vi "GUI Write Sequence Item Status.vi"(7 "status label":string="stat2", 8 "error in":errorcluster, 11 "sequence item":T1) -> (0 "error out":errorcluster, 3 "sequence item (copy)":T1)   [LabVIEW 2018]
doc: "Updates measurement status for each sequence item. Can generate error, but will exdcute even with input error."
uses:
  Meas Sequence Item.ctl
  Meas Sampling Configuration.ctl
  adc/ADC Trig Config.ctl
  adc/ADC Trig Mode Source.ctl
  adc/ADC Trig Coupling.ctl
  adc/ADC Trig Slope.ctl
  processing/QWTB/Meas Proc QWTB Algorithm Parameter Data.ctl
  varilib/SGUI Assign Multiple Strings With Tags By Label.vi
  varilib/varilib.lvlib
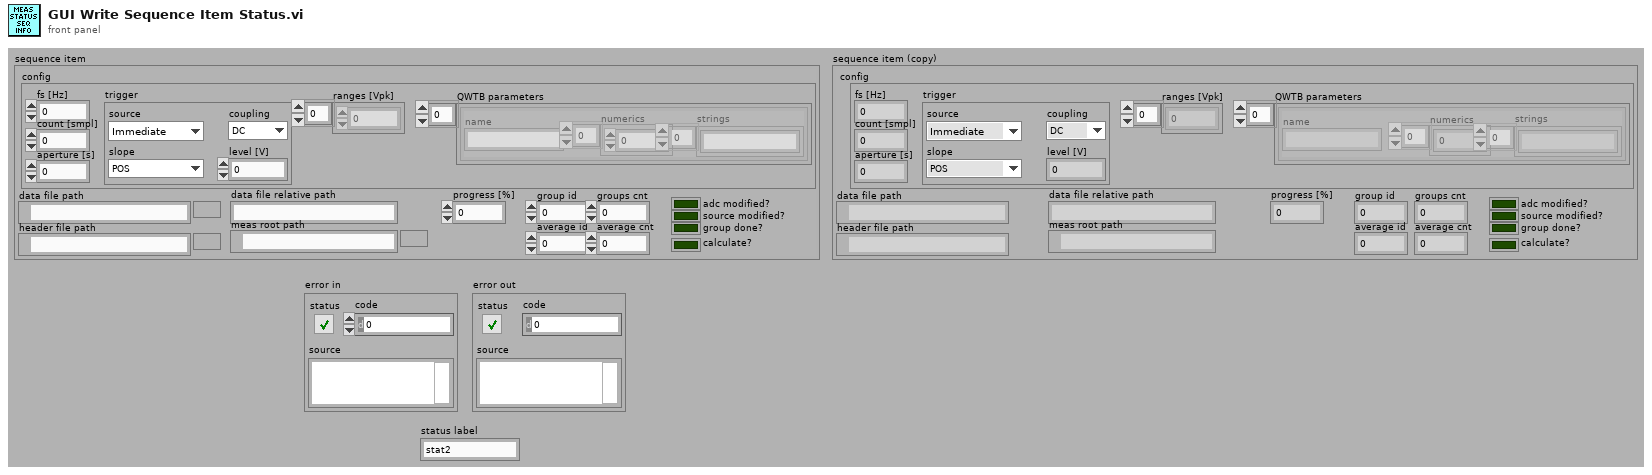
[diagram p1: front panel]
types:
  T1 = typedef "Meas Sequence Item.ctl" = cluster{"config":T2, "data file path":path, "header file path":path, "group id":i32, "average id":i32, "group done?":bool, "adc modified?":bool, "source modified?":bool, "progress [%]":dbl, "groups cnt":i32, "average cnt":i32, "data file relative path":string, "meas root path":path, "calculate?":bool}
  T2 = typedef "Meas Sampling Configuration.ctl" = cluster{"fs [Hz]":dbl, "count [smpl]":i64, "aperture [s]":dbl, "trigger":T3, "ranges [Vpk]":dbl[], "QWTB parameters":T7[]}
  T3 = typedef "ADC Trig Config.ctl" = cluster{"source":T4, "level [V]":dbl, "coupling":T5, "slope":T6}
  T4 = typedef "ADC Trig Mode Source.ctl" = enum16{"Immediate", "External", "Level"}
  T5 = typedef "ADC Trig Coupling.ctl" = enum16{"DC", "AC"}
  T6 = typedef "ADC Trig Slope.ctl" = enum16{"POS", "NEG"}
  T7 = typedef "Meas Proc QWTB Algorithm Parameter Data.ctl" = cluster{"name":string, "numerics":dbl[], "strings":string[]}
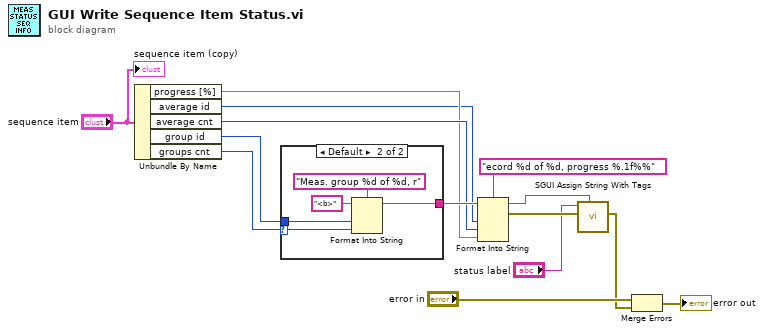
[diagram p0: block diagram]
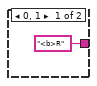
[diagram p2: hidden frame]
diagram:
  n1 = Unbundle By Name("sequence item") -> ("progress [%]"=w9:dbl, "average id"=w1:i32, "average cnt"=w10:i32, "group id"=w13:i32, "groups cnt"=w12:i32)
  n2 = case shown="Default" w12 {
    selector: w12 -> [_ w19]
    tunnel: w13 -> [_ w17]
    tunnel: ["<b>R" w18] -> w11
    frame 0, 1 {
    }
    frame Default {
      n3 = Format Into String(format string="Meas. group %d of %d, r", initial string="<b>", w17, w19) -> (resulting string=w18:string)  [unwired: 1 in, 1 out]
    }
  }
  n4 = Format Into String(format string="ecord %d of %d, progress %.1f%%", initial string=w11, w1, w10, w9) -> (resulting string=w7:string, error out=w8:errorcluster)  [unwired: 1 in]
  n5 = call-poly "SGUI Assign String With Tags.vi"("error in"=w8, "label(s) (empty)"="status label", "string (empty)"=w7) -> ("error out"=w3:errorcluster)  [unwired: 7 in, 1 out]
  n6 = Merge Errors("error in", w3) -> (→"error out":errorcluster)
  "sequence item (copy)" <- "sequence item"
